vi "cmd.vi"(7 "LabVIEW Web Service Request":refnum<class "Web Request.lvclass">) -> ()   [LabVIEW 2017]
uses:
  <vilib>/wsapi/Web Request.lvclass
  vsws_api/cmd.ctl
  vsws_api/vsws.lvlib
  <vilib>/NI_Real-Time Target Support.lvlib
panel:
  # "Use the Web Service Request input terminal to call the VIs on the Web Services palette. Do not remove it from the connector pane unless you don't need access to the palette."
  # "Each additional control wired to the connector pane will be available as an input in the URL. To include an indicator in terminal-mode output (the default setting), it must also be wired to the connector pane."
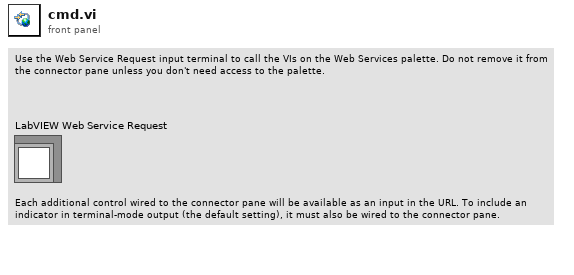
[diagram p1: front panel]
types:
  T1 = typedef "vsws.lvlib/cmd.ctl" = cluster{"postdata":string, "reponseQueue":refnum<queue>}
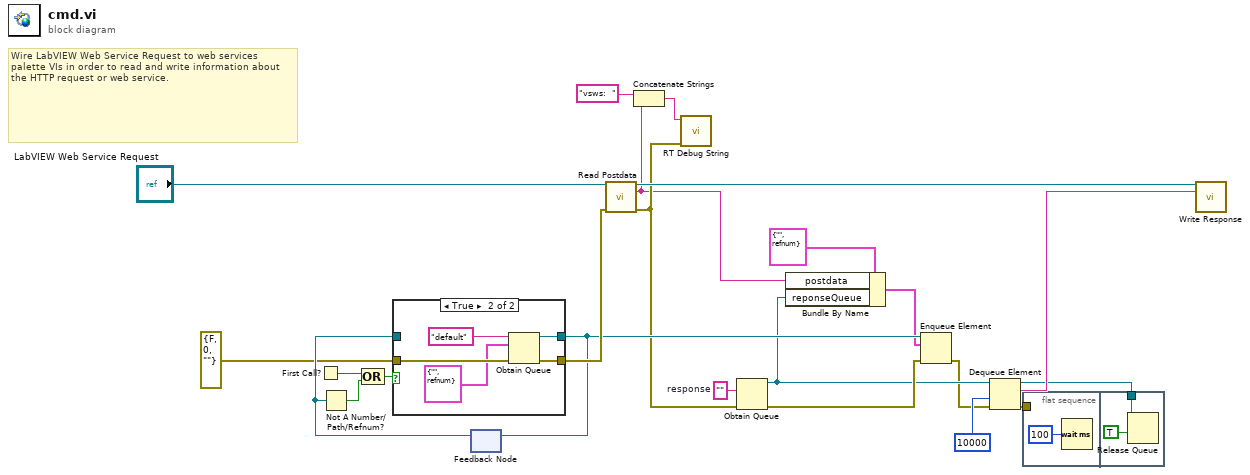
[diagram p0: block diagram]
diagram:
  w21 = ""  # response
  # "Wire LabVIEW Web Service Request to web services palette VIs in order to read and write information about the HTTP request or web service."
  n1 = First Call?() -> (First Call?: T/F=w19:bool)
  n2 = feedback #1() -> (w20:refnum<queue>)  [unwired: 1 in]
  n3 = Not A Number/Path/Refnum?(number/path/refnum=w20) -> (NaN/Path/Refnum?=w18:bool)
  n4 = Compound Arithmetic op=OR(w19, w18) -> (w17:bool)
  n5 = case shown="True" w17 {
    tunnel: errorcluster {"status"=FALSE, "code"=0, "source"=""} ("error in (no error)") -> [w24 w29]
    tunnel: [w25 w27] -> w13
    tunnel: w20 -> [w25 _]
    tunnel: [w24 w26] -> w14
    frame False {
    }
    frame True {
      n6 = Obtain Queue(name (unnamed)="default", element data type=T1 {"postdata"="", "reponseQueue"=refnum} ("cmd"), error in (no error)=w29) -> (queue out=w27:refnum<queue>, error out=w26:errorcluster)  [unwired: 2 in, 1 out]
    }
  }
  n7 = feedback-in #1(w13) -> ()
  n8 = call <vilib>:"Read Postdata.vi"("LabVIEW Web Service Request"="LabVIEW Web Service Request", "error in (no error)"=w14) -> ("LabVIEW Web Service Request out"=w22:refnum<class "Web Request.lvclass">, "postdata"=w4:string, "error out"=w6:errorcluster)  [unwired: 11 in]
  n9 = Concatenate Strings("vsws:  ", w4) -> (w3:string)
  n10 = call <vilib>:"RT Debug String.vi"("error in (no error)"=w6, "String to write"=w3) -> ()  [unwired: 9 in, 1 out]
  n11 = Obtain Queue(element data type=w21, error in (no error)=w6) -> (queue out=w10:refnum<queue>, error out=w11:errorcluster)  [unwired: 3 in, 1 out]
  n12 = Bundle By Name(cluster=T1 {"postdata"="", "reponseQueue"=refnum} ("cmd"), "postdata"=w4, "reponseQueue"=w10) -> (w12:T1)
  n13 = Enqueue Element(queue=w13, element=w12, error in (no error)=w11) -> (error out=w8:errorcluster)  [unwired: 1 in, 2 out]
  n14 = Dequeue Element(queue=w10, timeout in ms (-1)=10000, error in (no error)=w8) -> (queue out=w1:refnum<queue>, element=w7:string, error out=w2:errorcluster)  [unwired: 1 out]
  n15 = flat-sequence {
    tunnel: w2 -> [_]
    tunnel: w1 -> [w33]
    frame #0 {
      n16 = Wait (ms)(milliseconds to wait=u32 100) -> ()  [unwired: 1 out]
    }
    frame #1 {
      n17 = Release Queue(queue=w33, force destroy? (F)=TRUE) -> ()  [unwired: 1 in, 3 out]
    }
  }
  n18 = call <vilib>:"Write Response.vi"("LabVIEW Web Service Request"=w22, "response string"=w7) -> ()  [unwired: 12 in, 2 out]
